vi "DSF Configuration Cluster to File.vi"(8 "error in (no error)":errorcluster, 10 "framework configuration":T1, 11 "dsf configuration file path":path) -> (0 "error out":errorcluster, 3 "dsf configuration file path dup":path)   [LabVIEW 2017, in "DSF Core.lvlib" / "Configuration Session.lvclass"]
uses:
  Configuration Session.lvclass
  Typedefs/DSF Engine Framework Configuration.ctl
  Typedefs/DSF Engine Plugin Configuration.ctl
  Typedefs/DSF Timing Info.ctl
  Typedefs/DSF Engine Plugin Thread Configuration.ctl
  Typedefs/DSF Settings Info.ctl
  Typedefs/DSF Engine Transfer Group Configuration.ctl
  Typedefs/DSF Direction.ctl
  Typedefs/DSF Engine Transfer Configuration.ctl
  Typedefs/DSF Byte Order.ctl
  Typedefs/DSF Engine Channel Configuration.ctl
  Typedefs/DSF Data Type.ctl
  Typedefs/DSF Timeout Behavior.ctl
  Typedefs/DSF Plugin Info.ctl
  Typedefs/DSF Group Info.ctl
  Typedefs/DSF Transfer Info.ctl
  Typedefs/DSF Channel Info.ctl
  Write Channel.vi
  Add Channel.vi
  Write Transfer.vi
  Write Group.vi
  Write Plugin.vi
  DSF Core.lvlib
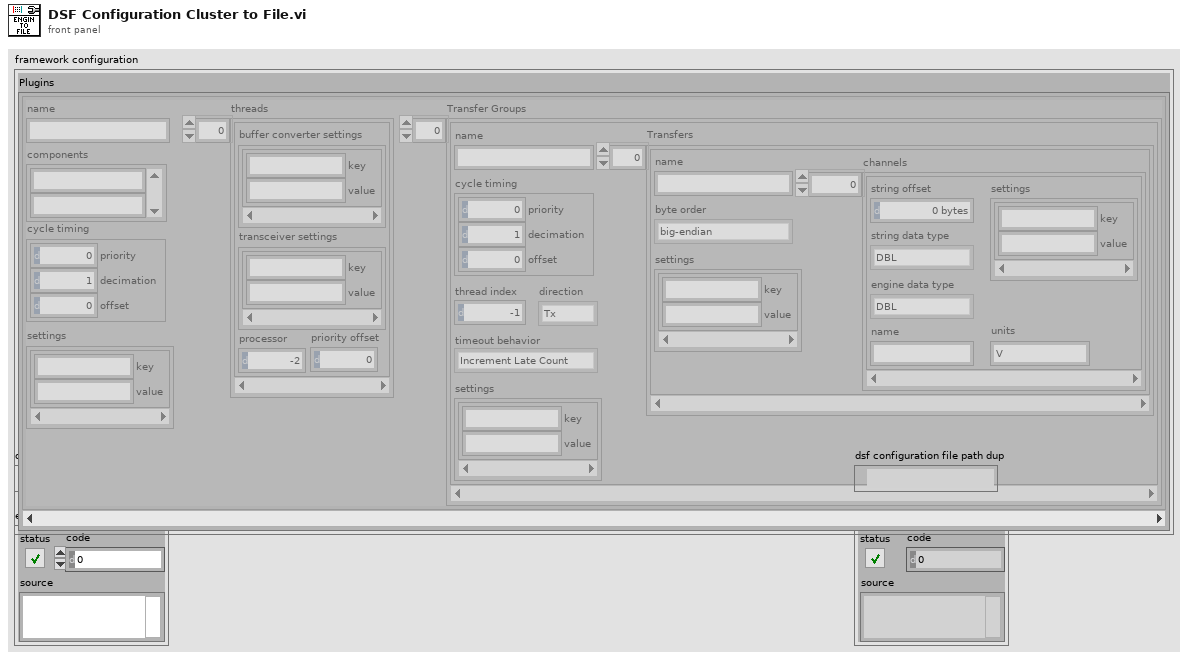
[diagram p1: front panel]
types:
  T1 = typedef "DSF Core.lvlib/DSF Engine Framework Configuration.ctl" = cluster{"Plugins":T2[]}
  T2 = typedef "DSF Core.lvlib/DSF Engine Plugin Configuration.ctl" = cluster{"name":string, "components":string[], "cycle timing":T3, "threads":T4[], "Transfer Groups":T6[], "settings":T5}
  T3 = typedef "DSF Core.lvlib/DSF Timing Info.ctl" = cluster{"priority":u64, "decimation":u64, "offset":u64}
  T4 = typedef "DSF Core.lvlib/DSF Engine Plugin Thread Configuration.ctl" = cluster{"buffer converter settings":T5, "transceiver settings":T5, "processor":i32, "priority offset":i16}
  T5 = typedef "DSF Core.lvlib/DSF Settings Info.ctl" = cluster{"key":string, "value":string}[]
  T6 = typedef "DSF Core.lvlib/DSF Engine Transfer Group Configuration.ctl" = cluster{"name":string, "direction":T7, "cycle timing":T3, "thread index":i32, "settings":T5, "Transfers":T8[], "timeout behavior":T12}
  T7 = typedef "DSF Core.lvlib/DSF Direction.ctl" = enum8{"Tx", "Rx"}
  T8 = typedef "DSF Core.lvlib/DSF Engine Transfer Configuration.ctl" = cluster{"name":string, "byte order":T9, "settings":T5, "channels":T10[]}
  T9 = typedef "DSF Core.lvlib/DSF Byte Order.ctl" = enum8{"big-endian", "little-endian"}
  T10 = typedef "DSF Core.lvlib/DSF Engine Channel Configuration.ctl" = cluster{"string offset":u64, "string data type":T11, "engine data type":T11, "name":string, "settings":T5, "units":string}
  T11 = typedef "DSF Core.lvlib/DSF Data Type.ctl" = enum8{"Bool", "SGL", "DBL", "I8", "I16", "I32", "I64", "U8", "U16", "U32", "U64"}
  T12 = typedef "DSF Core.lvlib/DSF Timeout Behavior.ctl" = enum8{"Increment Late Count", "Throw Error"}
  T13 = typedef "DSF Core.lvlib/DSF Plugin Info.ctl" = cluster{"components":string[], "timing":T3, "group ids":string[], "settings id":string, "threads":T4[]}
  T14 = typedef "DSF Core.lvlib/DSF Group Info.ctl" = cluster{"direction":T7, "timing":T3, "transfer ids":string[], "settings id":string, "thread":i32, "timeout behavior":T12}
  T15 = typedef "DSF Core.lvlib/DSF Transfer Info.ctl" = cluster{"byte order":T9, "channel ids":string[], "settings id":string}
  T16 = typedef "DSF Core.lvlib/DSF Channel Info.ctl" = cluster{"string buffer offset":u64, "string data type":T11, "engine data type":T11, "settings id":string, "units":string}
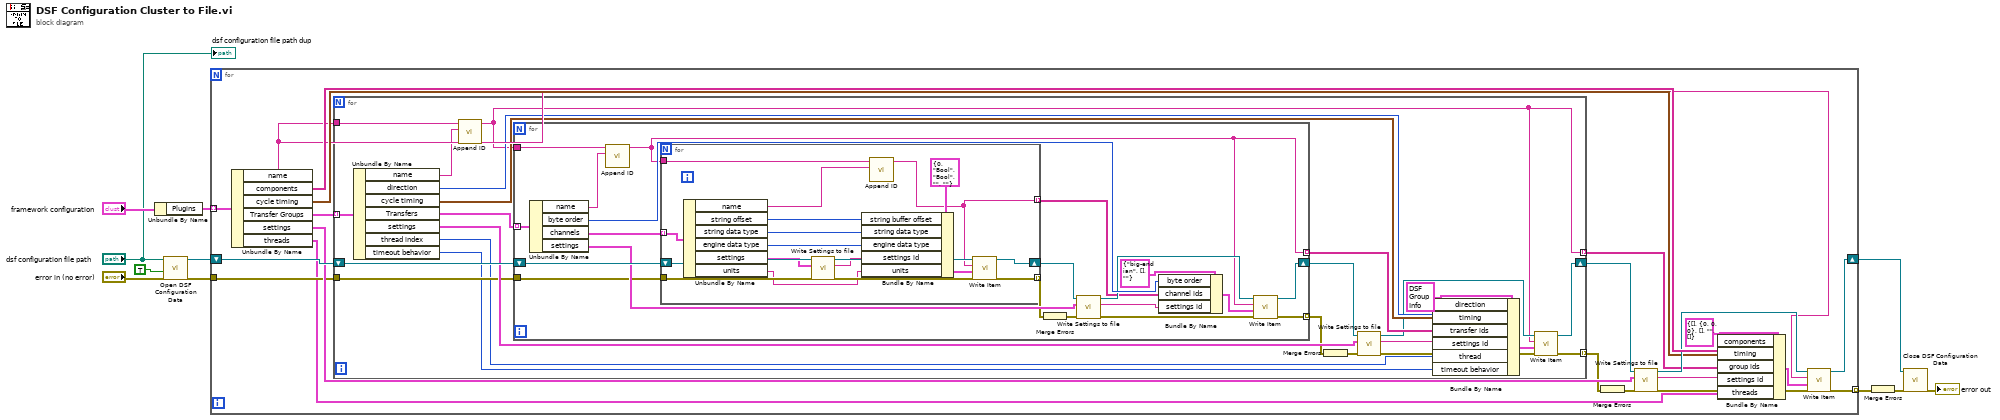
[diagram p0: block diagram]
diagram:
  n1 = Unbundle By Name("framework configuration") -> ("Plugins"=w8:T2[])
  n2 = call "Open DSF Configuration Data.vi"("error in (no error)"="error in (no error)", "replace if found? (F)"=TRUE, "dsf configuration file path"="dsf configuration file path") -> ("error out"=w5:errorcluster, "Configuration Session"=w7:refnum<class "Configuration Session.lvclass">)  [unwired: 4 in, 3 out]
  n3 = for {
    tunnel: w8 -> [w31] mode=indexing
    shift-right: [w25] -> w6
    shift-left: w7 -> [w26]
    tunnel: w5 -> [w19]
    tunnel: [w16] -> w4 mode=indexing
    n4 = Unbundle By Name(w31) -> ("name"=w12:string, "components"=w28:string[], "cycle timing"=w13:T3, "Transfer Groups"=w27:T6[], "settings"=w23:T5, "threads"=w14:T4[])
    n5 = for {
      tunnel: w27 -> [w54] mode=indexing
      shift-right: [w46] -> w21
      shift-left: w26 -> [w48]
      tunnel: [w33] -> w20 mode=indexing
      tunnel: w19 -> [w42]
      tunnel: [w41] -> w18 mode=indexing
      tunnel: w12 -> [w34]
      n6 = Unbundle By Name(w54) -> ("name"=w32:string, "direction"=w51:T7, "cycle timing"=w50:T3, "Transfers"=w49:T8[], "settings"=w45:T5, "thread index"=w37:i32, "timeout behavior"=w35:T12)
      n7 = call "Append ID.vi"("name"=w32, "initial id string (\"\")"=w34) -> ("appended id string"=w33:string)  [unwired: 9 in]
      n8 = for {
        tunnel: w49 -> [w74] mode=indexing
        shift-right: [w67] -> w47
        shift-left: w48 -> [w69]
        tunnel: [w55] -> w43 mode=indexing
        tunnel: w42 -> [w62]
        tunnel: [w59] -> w40 mode=indexing
        tunnel: w33 -> [w57]
        n9 = Unbundle By Name(w74) -> ("name"=w56:string, "byte order"=w72:T9, "channels"=w70:T10[], "settings"=w65:T5)
        n10 = call "Append ID.vi"("name"=w56, "initial id string (\"\")"=w57) -> ("appended id string"=w55:string)  [unwired: 9 in]
        n11 = for {
          tunnel: w70 -> [w92] mode=indexing
          shift-right: [w89] -> w68
          shift-left: w69 -> [w87]
          tunnel: [w78] -> w63 mode=indexing
          tunnel: w62 -> [w86]
          tunnel: [w88] -> w61 mode=indexing
          tunnel: w55 -> [w76]
          n12 = Unbundle By Name(w92) -> ("name"=w75:string, "string offset"=w79:u64, "string data type"=w80:T11, "engine data type"=w81:T11, "settings"=w85:T5, "units"=w77:string)
          n13 = call "Write Settings to file.vi"("error in (no error)"=w86, "settings"=w85, "Configuration Session in"=w87) -> ("error out"=w83:errorcluster, "settings id"=w82:string, "Configuration Session out"=w84:refnum<class "Configuration Session.lvclass">)  [unwired: 6 in]
          n14 = Bundle By Name(cluster=T16 {"string buffer offset"=0, "string data type"=enum."Bool", "engine data type"=enum."Bool", "settings id"="", "units"=""} ("values"), "string buffer offset"=w79, "string data type"=w80, "engine data type"=w81, "settings id"=w82, "units"=w77) -> (w90:T16)
          n15 = call "Append ID.vi"("name"=w75, "initial id string (\"\")"=w76) -> ("appended id string"=w78:string)  [unwired: 9 in]
          n16 = call-poly "Write Item.vi"("error in (no error)"=w83, "channel values"=w90, "id"=w78, "Configuration Session in"=w84) -> ("error out"=w88:errorcluster, "Configuration Session out"=w89:refnum<class "Configuration Session.lvclass">)  [unwired: 5 in, 1 out]
        }
        n17 = Merge Errors(w61) -> (w58:errorcluster)
        n18 = call "Write Settings to file.vi"("error in (no error)"=w58, "settings"=w65, "Configuration Session in"=w68) -> ("error out"=w60:errorcluster, "settings id"=w64:string, "Configuration Session out"=w66:refnum<class "Configuration Session.lvclass">)  [unwired: 6 in]
        n19 = Bundle By Name(cluster=T15 {"byte order"=enum."big-endian", "channel ids"=[], "settings id"=""} ("values"), "byte order"=w72, "channel ids"=w63, "settings id"=w64) -> (w71:T15)
        n20 = call-poly "Write Item.vi"("error in (no error)"=w60, "transfer values"=w71, "id"=w55, "Configuration Session in"=w66) -> ("error out"=w59:errorcluster, "Configuration Session out"=w67:refnum<class "Configuration Session.lvclass">)  [unwired: 5 in, 1 out]
      }
      n21 = Merge Errors(w40) -> (w38:errorcluster)
      n22 = call "Write Settings to file.vi"("error in (no error)"=w38, "settings"=w45, "Configuration Session in"=w47) -> ("error out"=w39:errorcluster, "settings id"=w44:string, "Configuration Session out"=w36:refnum<class "Configuration Session.lvclass">)  [unwired: 6 in]
      n23 = Bundle By Name(cluster=T14 {"direction"=enum."Tx", "timing"={"priority"=0, "decimation"=0, "offset"=0}, "transfer ids"=[], "settings id"="", "thread"=0, "timeout behavior"=enum."Increment Late Count"} ("group values"), "direction"=w51, "timing"=w50, "transfer ids"=w43, "settings id"=w44, "thread"=w37, "timeout behavior"=w35) -> (w52:T14)
      n24 = call-poly "Write Item.vi"("error in (no error)"=w39, "group values"=w52, "id"=w33, "Configuration Session in"=w36) -> ("error out"=w41:errorcluster, "Configuration Session out"=w46:refnum<class "Configuration Session.lvclass">)  [unwired: 5 in, 1 out]
    }
    n25 = Merge Errors(w18) -> (w15:errorcluster)
    n26 = call "Write Settings to file.vi"("error in (no error)"=w15, "settings"=w23, "Configuration Session in"=w21) -> ("error out"=w17:errorcluster, "settings id"=w24:string, "Configuration Session out"=w22:refnum<class "Configuration Session.lvclass">)  [unwired: 6 in]
    n27 = Bundle By Name(cluster=T13 {"components"=[], "timing"={"priority"=0, "decimation"=0, "offset"=0}, "group ids"=[], "settings id"="", "threads"=[]} ("plugin values"), "components"=w28, "timing"=w13, "group ids"=w20, "settings id"=w24, "threads"=w14) -> (w29:T13)
    n28 = call-poly "Write Item.vi"("error in (no error)"=w17, "plugin values"=w29, "id"=w12, "Configuration Session in"=w22) -> ("error out"=w16:errorcluster, "Configuration Session out"=w25:refnum<class "Configuration Session.lvclass">)  [unwired: 5 in, 1 out]
  }
  n29 = Merge Errors(w4) -> (w2:errorcluster)
  n30 = call "Close DSF Configuration Data.vi"("error in (no error)"=w2, "Configuration Session"=w6) -> ("error out"=→"error out":errorcluster)  [unwired: 8 in, 1 out]
  "dsf configuration file path dup" <- "dsf configuration file path"
